vi "logbtn.vi"() -> ()   [LabVIEW 2020]
uses:
  <vilib>/Utility/sysdir.llb/System Directory Type.ctl
panel:
  in  "stop":bool
  in  "C":bool
  in  "A":bool
  in  "B":bool
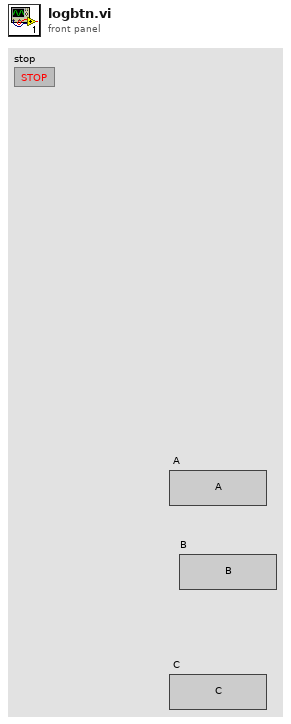
[diagram p1: front panel]
types:
  T1 = enum16{"open", "replace", "create", "open or create", "replace or create", "replace or create with confirmation"}
  T2 = typedef "System Directory Type.ctl" = i32
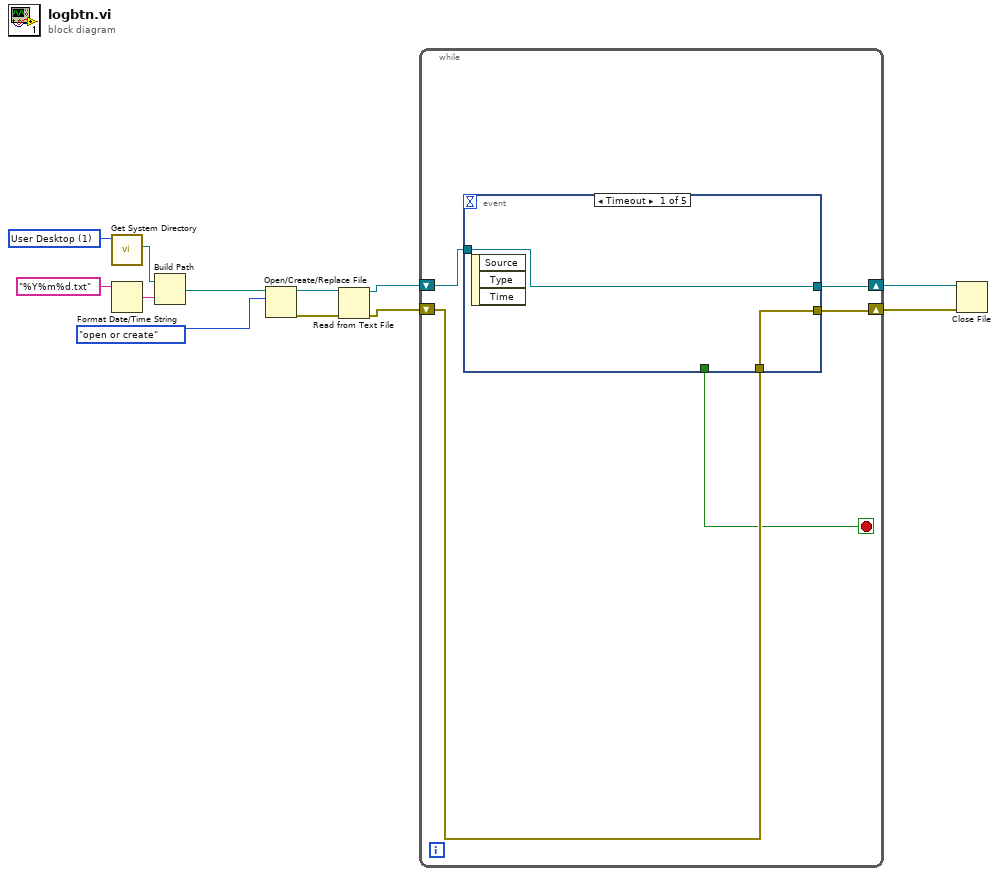
[diagram p0: block diagram]
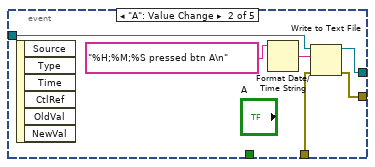
[diagram p2: hidden frame]
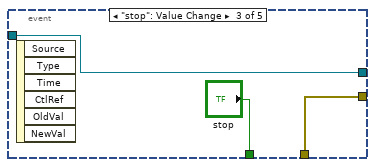
[diagram p3: hidden frame]
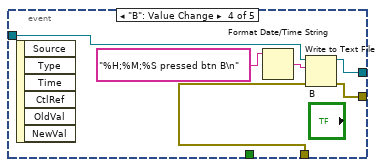
[diagram p4: hidden frame]
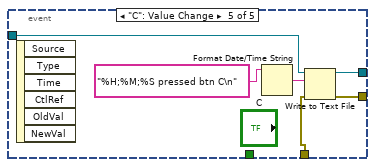
[diagram p5: hidden frame]
diagram:
  w12 = T2 1 items=["User Home"=0, "User Desktop"=1, "User Documents"=2, "User Application Data"=3, "User Preferences"=4, "User Temporary"=5, "Public Documents"=6, "Public Application Data"=7, "Public Preferences"=8, "Public Cache"=13, "System Core Libraries"=9, "System Installed Libraries"=10, "Application Files"=11, "Boot Volume Root"=12] ("system directory type")
  n1 = call <vilib>:"Get System Directory.vi"("system directory type"=w12) -> ("system directory"=w11:path)  [unwired: 10 in]
  n2 = Format Date/Time String(time format string (%c)="%Y%m%d.txt") -> (date/time string=w9:string)  [unwired: 2 in]
  n3 = Build Path(base path=w11, name or relative path=w9) -> (appended path=w7:path)
  n4 = Open/Create/Replace File(file path (use dialog)=w7, operation (0:open)=T1."open or create") -> (refnum out=w4:refnum<file>, error out=w1:errorcluster)  [unwired: 4 in, 1 out]
  n5 = Read from Text File(file (use dialog)=w4, error in=w1) -> (refnum out=w3:refnum<file>, error out=w2:errorcluster)  [unwired: 2 in, 2 out]
  n6 = while {
    shift-right: [w14] -> w6
    shift-left: w3 -> [w16]
    shift-right: [w15] -> w5
    shift-left: w2 -> [w17]
    stop <- w13 stop-if-true
    n7 = event shown="[0] Timeout" {
      selector: _ -> [_ _ _ _ _]
      dyn-events: _ -> [_ _ _ _ _]
      timeout: _ -> [_ _ _ _ _]
      tunnel: w16 -> [w19 w23 w27 w32 w37]
      tunnel: w17 -> [w18 w22 w26 w31 w38]
      tunnel: [w18 w21 w26 w29 w36] -> w15
      tunnel: [w19 w20 w27 w30 w35] -> w14
      tunnel: [_ _ "stop" _ _] -> w13
      event Timeout {
        n8 = event-data() -> ()  [unwired: 1 in, 3 out]
      }
      event "A": Value Change {
        n9 = event-data() -> ()  [unwired: 1 in, 6 out]
        n10 = Format Date/Time String(time format string (%c)="%H;%M;%S pressed btn A\n") -> (date/time string=w25:string)  [unwired: 2 in]
        n11 = Write to Text File(file (use dialog)=w23, text=w25, error in=w22) -> (refnum out=w20:refnum<file>, error out=w21:errorcluster)  [unwired: 1 in, 1 out]
      }
      event "stop": Value Change {
        n12 = event-data() -> ()  [unwired: 1 in, 6 out]
      }
      event "B": Value Change {
        n13 = event-data() -> ()  [unwired: 1 in, 6 out]
        n14 = Format Date/Time String(time format string (%c)="%H;%M;%S pressed btn B\n") -> (date/time string=w34:string)  [unwired: 2 in]
        n15 = Write to Text File(file (use dialog)=w32, text=w34, error in=w31) -> (refnum out=w30:refnum<file>, error out=w29:errorcluster)  [unwired: 1 in, 1 out]
      }
      event "C": Value Change {
        n16 = event-data() -> ()  [unwired: 1 in, 6 out]
        n17 = Format Date/Time String(time format string (%c)="%H;%M;%S pressed btn C\n") -> (date/time string=w40:string)  [unwired: 2 in]
        n18 = Write to Text File(file (use dialog)=w37, text=w40, error in=w38) -> (refnum out=w35:refnum<file>, error out=w36:errorcluster)  [unwired: 1 in, 1 out]
      }
    }
  }
  n19 = Close File(refnum=w6, error in=w5) -> ()  [unwired: 2 out]
